vi "Read 20T Magnet Field.vi"(7 "GPIB Adress":i16, 8 "error in (no error)":errorcluster) -> (0 "error out":errorcluster, 2 "Magnetic Field (Tesla)":dbl, 3 "Keithley Volts":dbl)   [LabVIEW 2015]
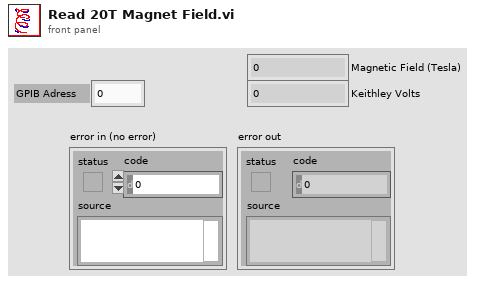
[diagram p1: front panel]
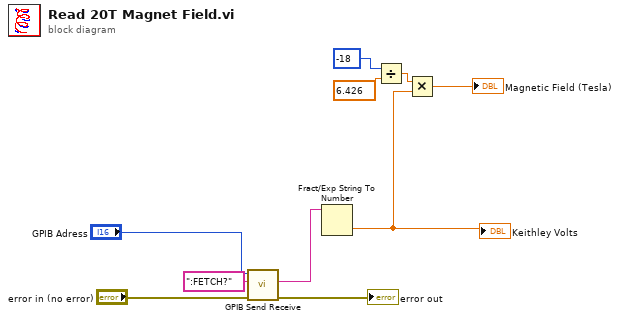
[diagram p0: block diagram]
diagram:
  n1 = call "GPIB Send Receive.vi"("error in (no error)"="error in (no error)", "data string in"=":FETCH?", "GPIB Adress"="GPIB Adress") -> ("error out"=→"error out":errorcluster, "data string out"=w6:string)  [unwired: 6 in, 1 out]
  n2 = Fract/Exp String To Number(string=w6) -> (number=w2:dbl)  [unwired: 3 in, 1 out]
  "Keithley Volts" <- w2
  n3 = Divide(x=-18, y=6.426) -> (x/y=w3:dbl)
  n4 = Multiply(x=w3, y=w2) -> (x*y=→"Magnetic Field (Tesla)":dbl)
